vi "Untitled 1.vi"() -> ()   [LabVIEW 2026]
uses:
  <vilib>/Analysis/5stat.llb/RMS (DBL).vi
  <vilib>/Analysis/baseanly.llb/Mean (DBL).vi
  <vilib>/Utility/file.llb/Read Delimited Spreadsheet (DBL).vi
  <vilib>/Analysis/NI_AALBase.lvlib
  <vilib>/Analysis/NI_AALPro.lvlib
panel:
  out "max value":dbl
  out "x-y":dbl
  out "x*y 2":dbl
  out "x*y":dbl
  out "log(x)":dbl
  out "x/y":dbl
  out "Vout":dbl[](array[numeric])
  out "subarray 2":dbl[](array[numeric])
  out "subarray":dbl[](array[numeric])
  out "all rows":dbl[][](array[numeric]) format="%#_6e"
  out "RMS Vout (V)":dbl
  out "RMS Vin (V)":dbl
  out "Mean Vout (V)":dbl
  out "Mean Vin (V)":dbl
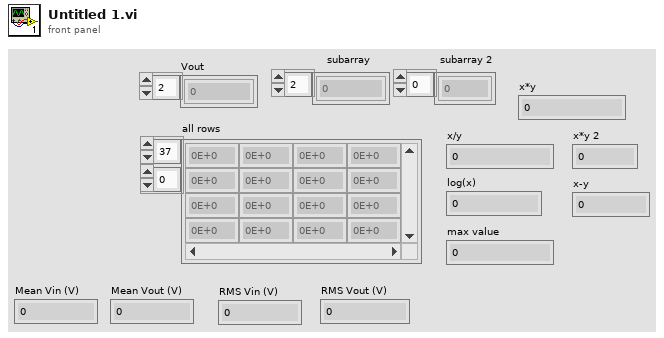
[diagram p1: front panel]
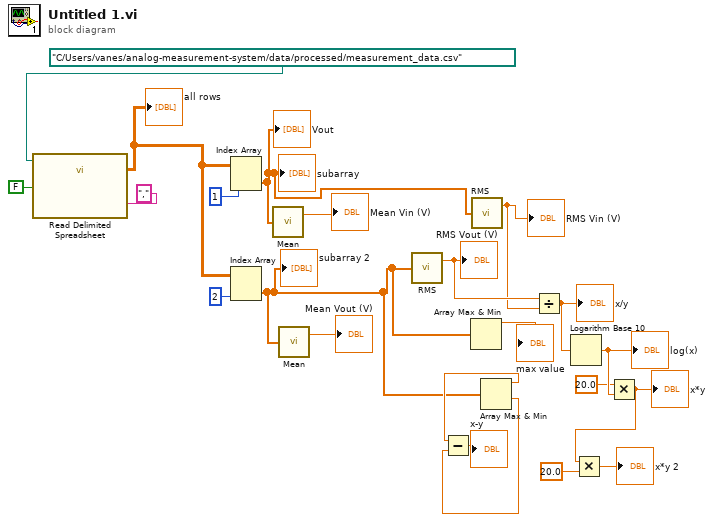
[diagram p0: block diagram]
diagram:
  n1 = call-poly <vilib>:"Read Delimited Spreadsheet.vi"("file path (dialog if empty)"=path "C:/Users/vanes/analog-measurement-system/data/processed/measurement_data.csv", "transpose? (F)"=FALSE, "delimiter (\\t)"=",") -> ("all rows"=w17:dbl[][])  [unwired: 7 in, 5 out]
  "all rows" <- w17
  n2 = Index Array(array=w17, index (col)=1 ("disabled index (col)")) -> (element=w14:dbl[])  [unwired: 1 in]
  "subarray" <- w14
  "Vout" <- w14
  n3 = Index Array(array=w17, index (col)=2) -> (element=w2:dbl[])  [unwired: 1 in]
  "subarray 2" <- w2
  n4 = call-poly <vilib>:"Mean.vi"("X"=w14) -> ("mean"=→"Mean Vin (V)":dbl)  [unwired: 1 out]
  n5 = call-poly <vilib>:"Mean.vi"("X"=w2) -> ("mean"=→"Mean Vout (V)":dbl)  [unwired: 1 out]
  n6 = call-poly <vilib>:"RMS.vi"("X"=w2) -> ("rms value"=w13:dbl)  [unwired: 1 out]
  "RMS Vout (V)" <- w13
  n7 = Array Max & Min(array=w2) -> (max value=→"max value":dbl)  [unwired: 3 out]
  n8 = call-poly <vilib>:"RMS.vi"("X"=w14) -> ("rms value"=w12:dbl)  [unwired: 1 out]
  "RMS Vin (V)" <- w12
  n9 = Array Max & Min(array=w2) -> (max value=w4:dbl, min value=w5:dbl)  [unwired: 2 out]
  n10 = Subtract(x=w4, y=w5) -> (x-y=→"x-y":dbl)
  n11 = Divide(x=w13, y=w12) -> (x/y=w11:dbl)
  "x/y" <- w11
  n12 = Logarithm Base 10(1:w11) -> (0:w10:dbl)
  "log(x)" <- w10
  n13 = Multiply(x=20.0, y=w10) -> (x*y=w8:dbl)
  "x*y" <- w8
  n14 = Multiply(x=w8, y=20.0) -> (x*y=→"x*y 2":dbl)
